vi "waypoint.vi"(6 "semaphore":T1, 7 "Motor Adress":T2(ring)=enum."3", 8 "error in (no error)":errorcluster, 10 "Profile Number":i32=123456, 11 "VISA ressource in":refnum<visa-resource-name>="COM1") -> (0 "error out":errorcluster={"status"=FALSE, "code"=1073676294, "source"="VISA Read in write_read.vi"}, 1 "Delta Steps":i32, 2 "Log File":string, 3 "VISA ressource out":refnum<visa-resource-name>)   [LabVIEW 2013]
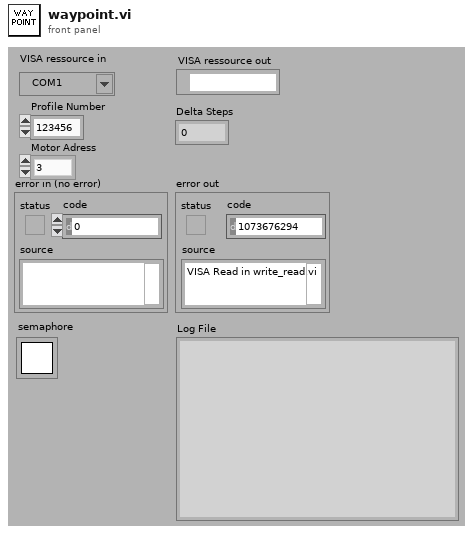
[diagram p1: front panel]
types:
  T1 = typedef "Semaphore RefNum" = refnum<k1>
  T2 = enum16{"All", "1", "2", "3", "4", "5", "6", "7", "8"}
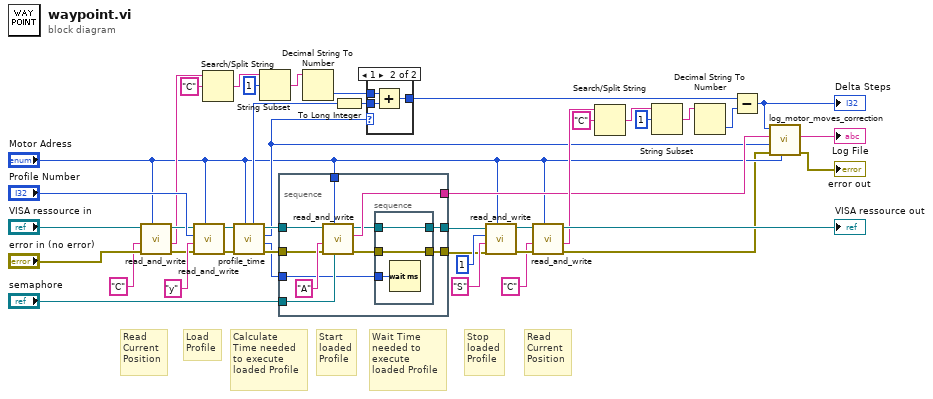
[diagram p0: block diagram]
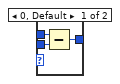
[diagram p2: hidden frame]
diagram:
  # "Wait Time\nneeded to\nexecute\nloaded Profile"
  # "Read\nCurrent\nPosition"
  # "Stop\nloaded\nProfile"
  # "Start\nloaded\nProfile"
  # "Calculate\nTime needed\nto execute\nloaded Profile"
  # "Load\nProfile"
  # "Read\nCurrent\nPosition"
  n1 = call "read_and_write.vi"("Motor Adress"="Motor Adress", "error in (no error)"="error in (no error)", "Command"="C", "VISA ressource in"="VISA ressource in") -> ("error out"=w37:errorcluster, "Answer"=w23:string, "VISA ressource out"=w36:refnum<visa-resource-name>)  [unwired: 4 in, 1 out]
  n2 = call "read_and_write.vi"("Motor Adress"="Motor Adress", "error in (no error)"=w37, "Command"="y", "value"="Profile Number", "VISA ressource in"=w36) -> ("error out"=w33:errorcluster, "VISA ressource out"=w32:refnum<visa-resource-name>)  [unwired: 3 in, 2 out]
  n3 = Search/Split String(string=w23, search string/char (-)="C") -> (match + rest of string=w21:string)  [unwired: 1 in, 2 out]
  n4 = call "profile_time.vi"("Motor Adress"="Motor Adress", "error in (no error)"=w33, "VISA ressource in"=w32) -> ("error out"=w30:errorcluster, "profile time (in ms)"=w8:u32, "direction"=w4:i32, "VISA ressource out"=w31:refnum<visa-resource-name>, "steps"=w11:u32)  [unwired: 4 in]
  n5 = String Subset(string=w21, offset (0)=1) -> (substring=w19:string)  [unwired: 1 in]
  n6 = stacked-sequence {
    tunnel: w31 -> [w53]
    tunnel: w30 -> [w52]
    tunnel: [w51] -> w5
    tunnel: "semaphore" -> [w50]
    tunnel: "Motor Adress" -> [w49]
    tunnel: [w46] -> w29
    tunnel: [w45] -> w28
    tunnel: w8 -> [w44]
    frame #0 {
      n7 = call "read_and_write.vi"("semaphore"=w50, "Motor Adress"=w49, "error in (no error)"=w52, "Command"="A", "VISA ressource in"=w53) -> ("error out"=w47:errorcluster, "Log File (global)"=w51:string, "VISA ressource out"=w48:refnum<visa-resource-name>)  [unwired: 3 in, 1 out]
      n8 = stacked-sequence {
        tunnel: w48 -> [w56]
        tunnel: w47 -> [w57]
        tunnel: [w57] -> w45
        tunnel: [w56] -> w46
        tunnel: w44 -> [w55]
        frame #0 {
          n9 = Wait (ms)(milliseconds to wait=w55) -> ()  [unwired: 1 out]
        }
      }
    }
  }
  n10 = Decimal String To Number(string=w19) -> (number=w12:i32)  [unwired: 2 in, 1 out]
  n11 = To Long Integer(number=w11) -> (32bit integer=w10:i32)
  n12 = case shown="1" w4 {
    tunnel: w12 -> [w60 w63]
    tunnel: w10 -> [w59 w62]
    tunnel: [w58 w61] -> w9
    frame 0, Default {
      n13 = Subtract(x=w60, y=w59) -> (x-y=w58:i32)
    }
    frame 1 {
      n14 = Add(x=w63, y=w62) -> (x+y=w61:i32)
    }
  }
  n15 = call "read_and_write.vi"("Motor Adress"="Motor Adress", "error in (no error)"=w28, "Command"="S", "value"=1, "VISA ressource in"=w29) -> ("error out"=w27:errorcluster, "VISA ressource out"=w26:refnum<visa-resource-name>)  [unwired: 3 in, 2 out]
  n16 = call "read_and_write.vi"("Motor Adress"="Motor Adress", "error in (no error)"=w27, "Command"="C", "VISA ressource in"=w26) -> ("error out"=w2:errorcluster, "Answer"=w14:string, "VISA ressource out"=→"VISA ressource out":refnum<visa-resource-name>)  [unwired: 4 in, 1 out]
  n17 = Search/Split String(string=w14, search string/char (-)="C") -> (match + rest of string=w16:string)  [unwired: 1 in, 2 out]
  n18 = String Subset(string=w16, offset (0)=1) -> (substring=w18:string)  [unwired: 1 in]
  n19 = Decimal String To Number(string=w18) -> (number=w13:i32)  [unwired: 2 in, 1 out]
  n20 = Subtract(x=w9, y=w13) -> (x-y=w7:i32)
  "Delta Steps" <- w7
  n21 = call "log_motor_moves_correction.vi"("Motor Adress"="Motor Adress", "error in"=w2, "Direction"=w4, "Log File IN"=w5, "Delta Steps"=w7) -> ("error out"=→"error out":errorcluster, "Log File OUT"=→"Log File":string)  [unwired: 5 in]
